vi "CAN UDS Request.vi"(6 "DataLen":i32, 7 "pReqData":u8[](array[numeric])=array[4097 elements], 8 "error in (no error)":errorcluster, 9 "pUDSAddr":T1, 10 "CANIndex":u8, 11 "DevHandle":i32) -> (0 "error out":errorcluster, 1 "pUDSAddr out":T1, 3 "function return":i32, 5 "pReqData out":u8[](array[numeric]))   [LabVIEW 2010, in "can_uds.lvlib"]
doc: "int WINAPI CAN_UDS_Request(int DevHandle,unsigned char CANIndex,CAN_UDS_ADDR *pUDSAddr,unsigned char *pReqData,int DataLen);"
uses:
  can_uds.lvlib
  USB2XXX/trunk/USB2XXX/USB2XXX/vs2010/Release/USB2XXX.dll
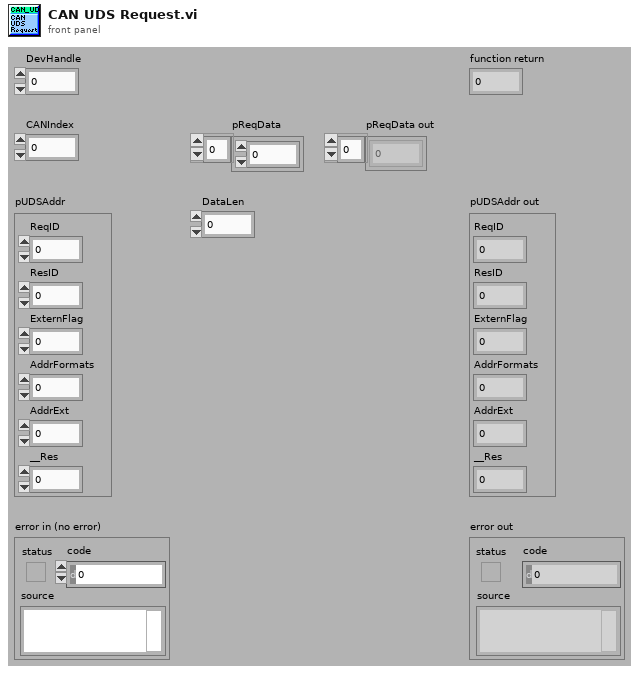
[diagram p1: front panel]
types:
  T1 = cluster{"ReqID":u32, "ResID":u32, "ExternFlag":u8, "AddrFormats":u8, "AddrExt":u8, "__Res":u8}
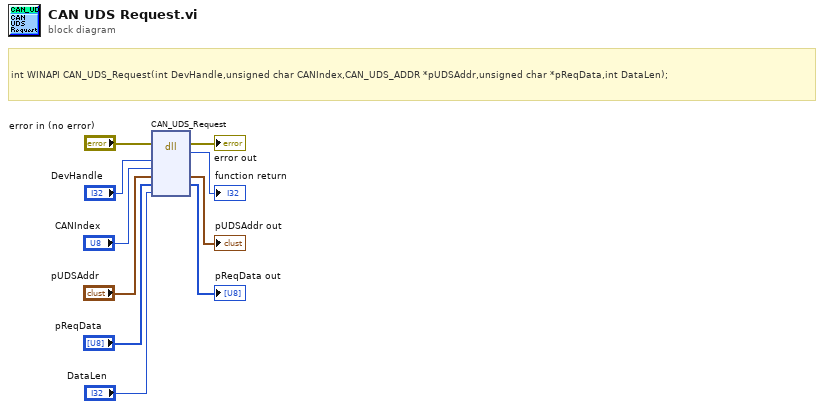
[diagram p0: block diagram]
diagram:
  # "int WINAPI CAN_UDS_Request(int DevHandle,unsigned char CANIndex,CAN_UDS_ADDR *pUDSAddr,unsigned char *pReqData,int DataLen);"
  n1 = dll-call lib="E:/OtherWork/STM32/USB2XXX/trunk/USB2XXX/USB2XXX/vs2010/Release/USB2XXX.*" fn="CAN_UDS_Request"(error in="error in (no error)", "DevHandle"="DevHandle", "CANIndex"="CANIndex", "pUDSAddr"="pUDSAddr", "pReqData"="pReqData", "DataLen"="DataLen") -> (error out=→"error out":errorcluster, →"function return":i32, "pUDSAddr"=→"pUDSAddr out":T1, "pReqData"=→"pReqData out":u8[])  [unwired: 5 in, 1 out]
